vi "Set All.vi"(8 "error in (no error)":errorcluster, 9 "Camera Settings":T1={"Exposure Time (ms)"=100.0, "Binning"=enum."2x2", "Scan Mode"=-1, "Frames to Acquire"=1000.0, "Pixel Correction"=FALSE, "Frames to Skip"=1, "File Path"=path "", "Duty cycle"=1.0, "ALEX"=FALSE, "Shutter Enable"=[], "fluidics trigger frame"=0, "Bit Depth"=16, "Image Width (px)"=0, "Image Height (px)"=0, "Horizontal Offset (px)"=0, "Vertical Offset (px)"=0} {"fluidics trigger frame" max=60000 step=1; "Exposure Time (ms)" min=1.0 max=10000.0 step=1.0}, 10 "Streaming?":bool, 11 "Synchronization Device in":refnum<class "NI DAQ.lvclass">) -> (0 "error out":errorcluster, 3 "Synchronization Device out":refnum<class "NI DAQ.lvclass">)   [LabVIEW 2023, in "NI DAQ.lvlib" / "NI DAQ.lvclass"]
uses:
  NI DAQ.lvclass
  Resources/Type Defs/Camera Settings.ctl
  NI DAQ.lvclass/NI DAQ.ctl
  Resources/GLOBAL/GLOBAL Experiment Metadata.vi
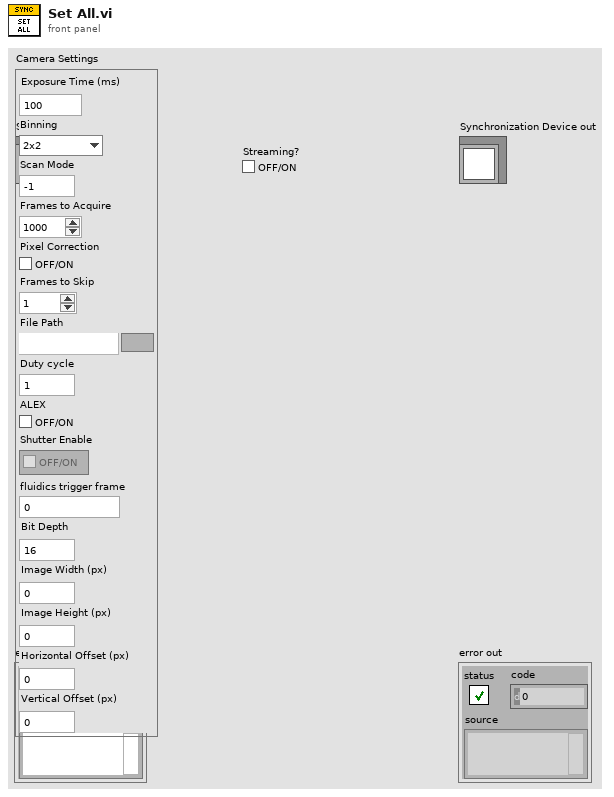
[diagram p1: front panel]
types:
  T1 = typedef "Camera Settings.ctl" = cluster{"Exposure Time (ms)":dbl, "Binning":enum16{"1x1", "2x2", "4x4"}, "Scan Mode":i32, "Frames to Acquire":dbl, "Pixel Correction":bool, "Frames to Skip":u32, "File Path":path, "Duty cycle":dbl, "ALEX":bool, "Shutter Enable":bool[], "fluidics trigger frame":u16, "Bit Depth":u16, "Image Width (px)":u16, "Image Height (px)":u16, "Horizontal Offset (px)":u16, "Vertical Offset (px)":u16}
  T2 = cluster{"Shutter Enable":bool[], "Duty Cycle":dbl, "Wavelengths":dbl[], "ALEX?":bool}
  T3 = typedef "sync device settings.ctl" = cluster{"Interval (ms)":dbl, "ALEX":bool, "Shutter Enable":bool[], "Stream":bool, "Duty Cycle":dbl, "fluidics trigger frame":u16, "Frames to Skip":u32}
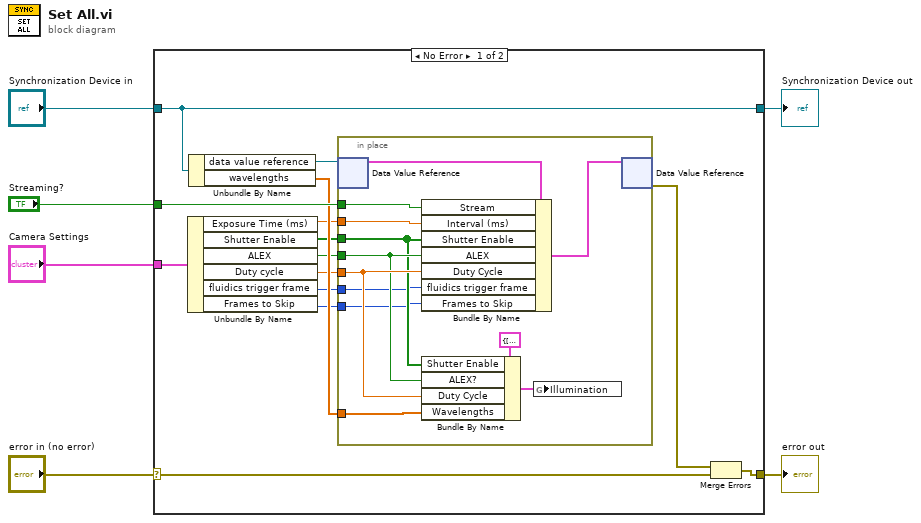
[diagram p0: block diagram]
diagram:
  n1 = case shown="No Error" "error in (no error)" {
    selector: "error in (no error)" -> [w18 w34]
    tunnel: [w19 w34] -> w5
    tunnel: [w20 w33] -> w3
    tunnel: "Synchronization Device in" -> [w20 w33]
    tunnel: "Streaming?" -> [w16 _]
    tunnel: "Camera Settings" -> [w13 _]
    frame No Error {
      n2 = Unbundle By Name(w13) -> ("Exposure Time (ms)"=w12:dbl, "Shutter Enable"=w11:bool[], "ALEX"=w10:bool, "Duty cycle"=w9:dbl, "fluidics trigger frame"=w8:u16, "Frames to Skip"=w7:u32)
      n3 = Unbundle By Name(w20) -> ("data value reference"=w17:refnum<data-value>, "wavelengths"=w14:dbl[])
      n4 = in-place {
        in-place-border: w16 -> [w31]
        in-place-border: w14 -> [w27]
        in-place-border: w12 -> [w26]
        in-place-border: w9 -> [w25]
        in-place-border: w10 -> [w24]
        in-place-border: w11 -> [w23]
        in-place-border: w8 -> [w22]
        in-place-border: w7 -> [w21]
        n5 = in-place-dvr #1(w17) -> (w30:T3)  [unwired: 1 out]
        n6 = Bundle By Name(cluster=w30, "Stream"=w31, "Interval (ms)"=w26, "Shutter Enable"=w23, "ALEX"=w24, "Duty Cycle"=w25, "fluidics trigger frame"=w22, "Frames to Skip"=w21) -> (w32:T3)
        n7 = Bundle By Name(cluster=T2 {"Shutter Enable"=[], "Duty Cycle"=0.0, "Wavelengths"=[], "ALEX?"=FALSE} ("Cluster"), "Shutter Enable"=w23, "ALEX?"=w24, "Duty Cycle"=w25, "Wavelengths"=w27) -> (w29:T2)
        n8 = global write "GLOBAL Experiment Metadata.vi" "Illumination"(w29) -> ()
        n9 = in-place-dvr #1(w32) -> (w15:errorcluster)  [unwired: 1 out]
      }
      n10 = Merge Errors(w15, w18) -> (w19:errorcluster)
    }
    frame Error {
    }
  }
  "error out" <- w5
  "Synchronization Device out" <- w3
